vi "Config - Update.vi"(8 "error in (no error)":errorcluster, 10 "Data Record":T1, 11 "Data Records":T1[](array[typedef])) -> (0 "error out":errorcluster, 3 "Data Records":T1[](array[typedef]))   [LabVIEW 2017]
doc: "Updates current values in Data Records Array\nwith new values from input control Data Record"
uses:
  Controls/Config Data Record.ctl
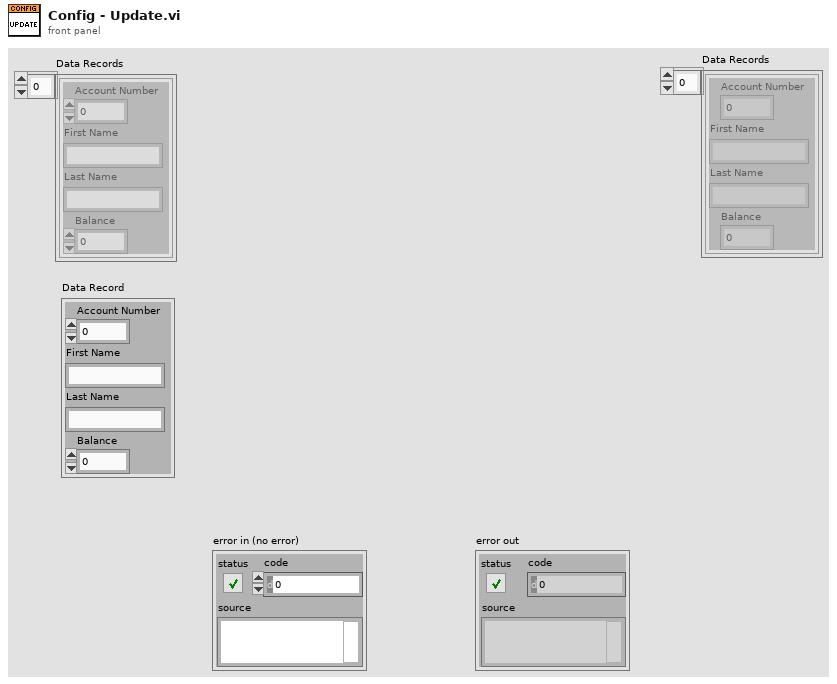
[diagram p1: front panel]
types:
  T1 = typedef "Config Data Record.ctl" = cluster{"Account Number":u32, "First Name":string, "Last Name":string, "Balance":dbl}
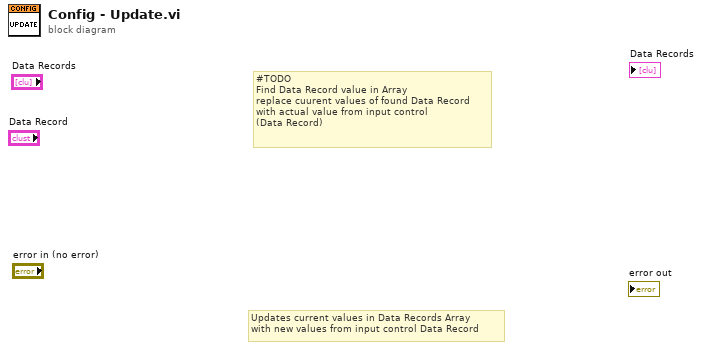
[diagram p0: block diagram]
diagram:
  # "#TODO\nFind Data Record value in Array\nreplace cuurent values of found Data Record\nwith actual value from input control\n(Data Record)"
  # "Updates current values in Data Records Array\nwith new values from input control Data Record"
